vi "INTERFAZ.vi"() -> ()   [LabVIEW 2017]
uses:
  <vilib>/Instr/_visa.llb/VISA Configure Serial Port (Instr).vi
panel:
  out "V1 / V2":dbl
  out "Q 2  [m3/s] 2":dbl
  out "V2  [m3/s] 2":dbl
  out "V1  [m/s] 2":dbl
  out "Q 1 [m3/s] 2":dbl
  out "Q 2  [m3/s]":dbl
  out "P2 [Pa]":dbl
  out "P1  [Pa]":dbl
  out "V2  [m/s]":dbl
  out "V1  [m/s]":dbl
  out "Q 1 [m3/s]":dbl
  out "P1 / P2":dbl
  in  "ELECTROVALVULA":bool
  out "BYTE 7":u8
  out "BYTE 6":u8
  out "BYTE 5":u8
  out "BYTE 4":u8
  out "BYTE 3":u8
  out "BYTE 2":u8
  out "BYTE 1":u8
  out "BYTE0":u8
  in  "PUERTO SERIE ARDUINO":refnum<visa-resource-name>
  in  "STOP":bool
  out "CAUDAL 2 [L/min]":dbl(knob) scale=0.0..800.0
  out "CAUDAL 1 [L/min]":dbl(knob) scale=0.0..800.0
  out "PRESION 1 [PSI]":dbl(knob) scale=10.0..80.0
  out "PRESION 2 [PSI]":dbl(knob) scale=10.0..80.0
  # "PROYECTO TUBO VENTURI - DEMOSTRACION EXPERIMENTAL"
  # "ERROR %"
  # "VALORES EXPERIMENTALES"
  # "VALORES TEORICOS"
  # "RELACIONES"
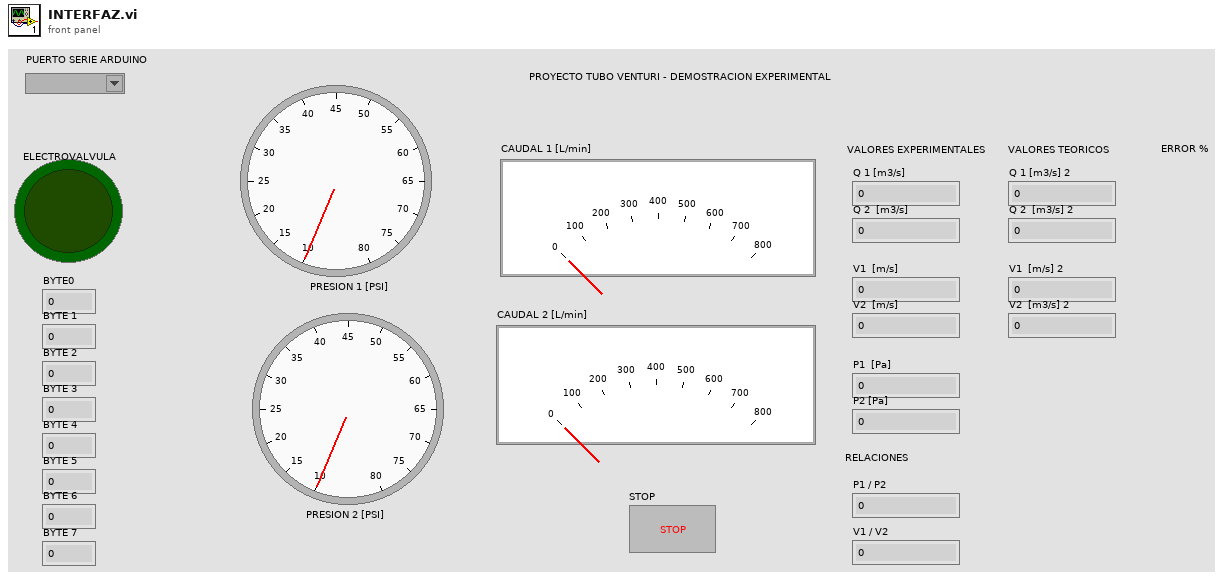
[diagram p1: front panel]
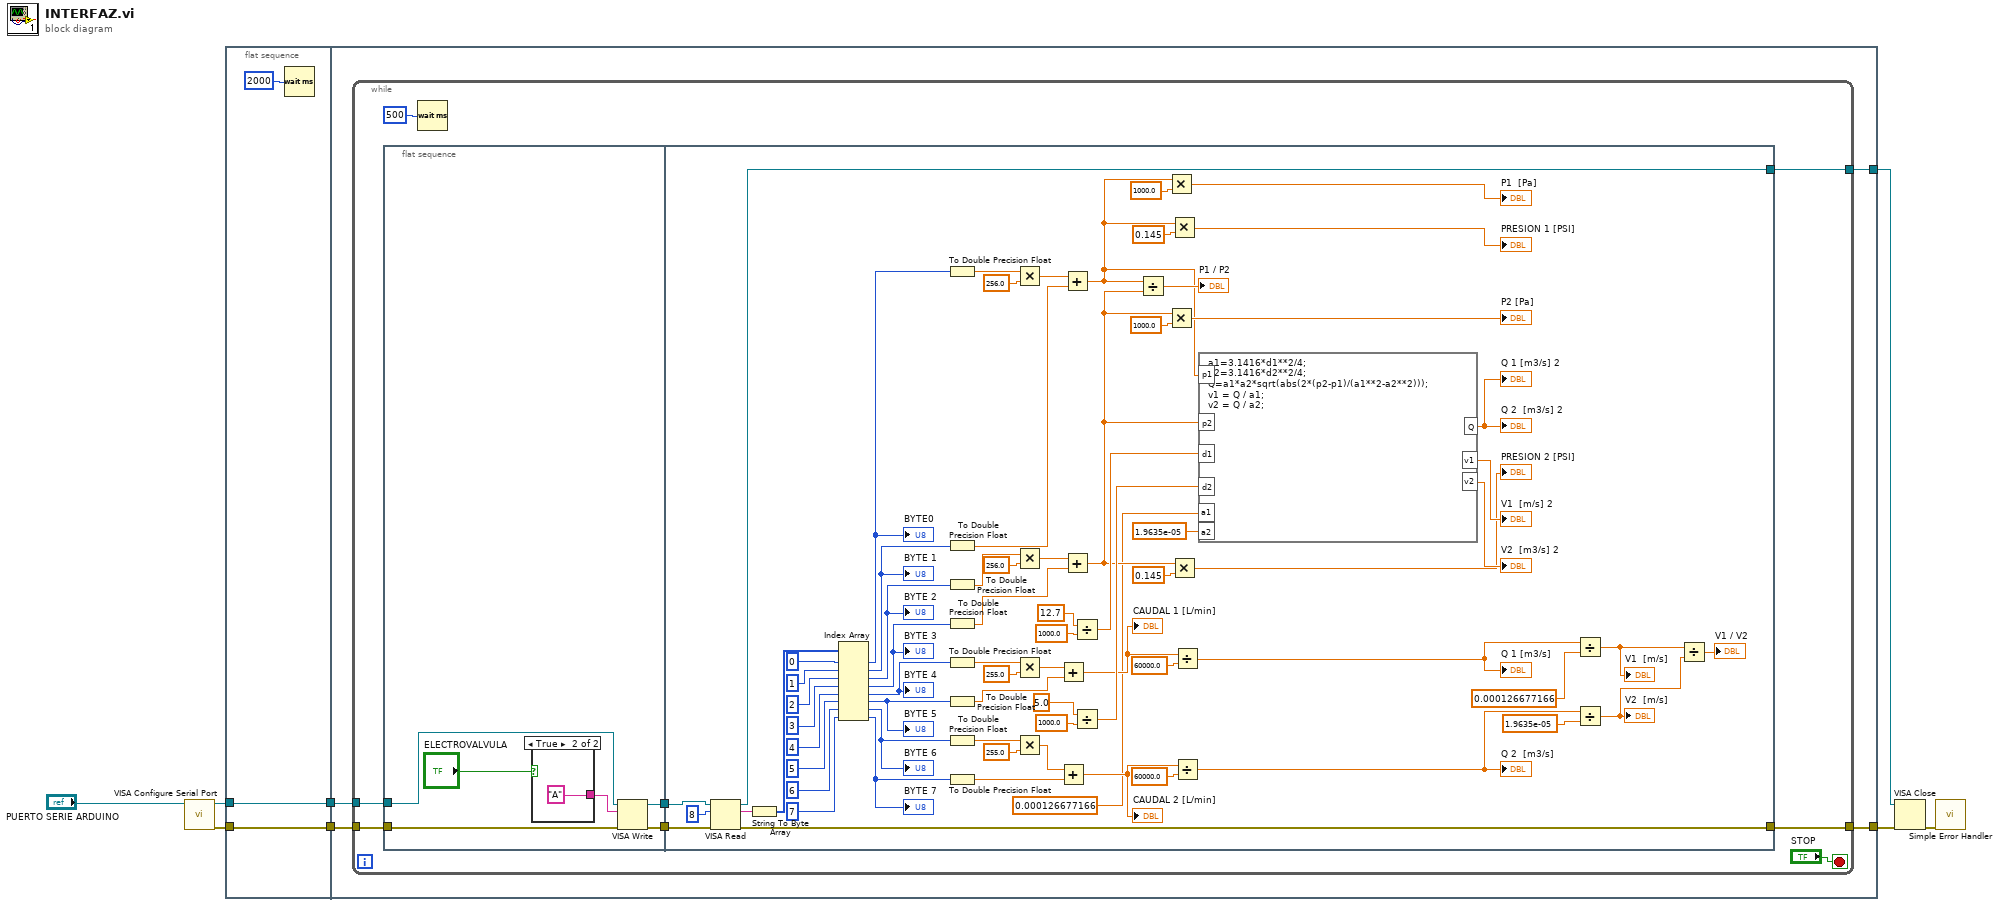
[diagram p0: block diagram]
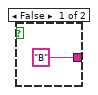
[diagram p2: hidden frame]
diagram:
  n1 = call-poly "VISA Configure Serial Port"("VISA resource name"="PUERTO SERIE ARDUINO") -> ("VISA resource name out"=w6:refnum<visa-resource-name>, "error out"=w4:errorcluster)  [unwired: 13 in]
  n2 = flat-sequence {
    tunnel: [w10] -> w7
    tunnel: w6 -> [w10]
    tunnel: [w9] -> w5
    tunnel: w4 -> [w9]
    tunnel: w7 -> [w14]
    tunnel: w5 -> [w15]
    tunnel: [w13] -> w3
    tunnel: [w12] -> w2
    frame #0 {
      n3 = Wait (ms)(milliseconds to wait=u32 2000) -> ()  [unwired: 1 out]
    }
    frame #1 {
      n4 = while {
        tunnel: w15 -> [w22]
        tunnel: w14 -> [w21]
        tunnel: [w18] -> w13
        tunnel: [w17] -> w12
        stop <- "STOP" stop-if-true
        n5 = flat-sequence {
          tunnel: w22 -> [w29]
          tunnel: w21 -> [w28]
          tunnel: [w27] -> w20
          tunnel: [w26] -> w19
          tunnel: w20 -> [w103]
          tunnel: w19 -> [w102]
          tunnel: [w96] -> w18
          tunnel: [w95] -> w17
          frame #0 {
            n6 = case shown="True" "ELECTROVALVULA" {
              tunnel: ["B" ("write buffer") "A" ("write buffer")] -> w24
              frame False {
              }
              frame True {
              }
            }
            n7 = VISA Write(VISA resource name=w28, write buffer=w24, error in (no error)=w29) -> (VISA resource name out=w27:refnum<visa-resource-name>, error out=w26:errorcluster)  [unwired: 1 out]
          }
          frame #1 {
            n8 = VISA Read(VISA resource name=w103, byte count=u32 8, error in (no error)=w102) -> (VISA resource name out=w96:refnum<visa-resource-name>, read buffer=w100:string, error out=w95:errorcluster)  [unwired: 1 out]
            n9 = String To Byte Array(string=w100) -> (unsigned byte array=w99:u8[])
            n10 = Index Array(array=w99, index #1=0 ("index"), index #2=1 ("index"), index #3=2 ("index"), index #4=3 ("index"), index #5=4 ("index"), index #6=5 ("index"), index #7=6 ("index"), index #8=7 ("index")) -> (element #1=w85:u8, element #2=w83:u8, element #3=w78:u8, element #4=w77:u8, element #5=w72:u8, element #6=w71:u8, element #7=w66:u8, element #8=w65:u8)
            "BYTE0" <- w85
            "BYTE 1" <- w83
            "BYTE 2" <- w78
            "BYTE 3" <- w77
            "BYTE 4" <- w72
            "BYTE 5" <- w71
            "BYTE 6" <- w66
            "BYTE 7" <- w65
            n11 = To Double Precision Float(number=w85) -> (double precision float=w86:dbl)
            n12 = To Double Precision Float(number=w83) -> (double precision float=w84:dbl)
            n13 = To Double Precision Float(number=w78) -> (double precision float=w80:dbl)
            n14 = To Double Precision Float(number=w77) -> (double precision float=w79:dbl)
            n15 = To Double Precision Float(number=w72) -> (double precision float=w74:dbl)
            n16 = To Double Precision Float(number=w71) -> (double precision float=w73:dbl)
            n17 = To Double Precision Float(number=w66) -> (double precision float=w68:dbl)
            n18 = To Double Precision Float(number=w65) -> (double precision float=w67:dbl)
            n19 = Multiply(x=w86, y=256.0) -> (x*y=w87:dbl)
            n20 = Multiply(x=w80, y=256.0) -> (x*y=w81:dbl)
            n21 = Multiply(x=w74, y=255.0) -> (x*y=w75:dbl)
            n22 = Multiply(x=w68, y=255.0) -> (x*y=w69:dbl)
            n23 = Add(x=w75, y=w73) -> (x+y=w53:dbl)
            "CAUDAL 1 [L/min]" <- w53
            n24 = Add(x=w69, y=w67) -> (x+y=w50:dbl)
            "CAUDAL 2 [L/min]" <- w50
            n25 = Add(x=w87, y=w84) -> (x+y=w41:dbl)
            n26 = Add(x=w81, y=w79) -> (x+y=w45:dbl)
            n27 = Divide(x=12.7 ("input variable"), y=1000.0) -> (x/y=w59:dbl)
            n28 = Divide(x=5.0 ("input variable"), y=1000.0) -> (x/y=w58:dbl)
            n29 = Divide(x=w41, y=w45) -> (x/y=→"P1 / P2":dbl)
            n30 = Multiply(x=w41, y=1000.0) -> (x*y=→"P1  [Pa]":dbl)
            n31 = Multiply(x=w45, y=1000.0) -> (x*y=→"P2 [Pa]":dbl)
            n32 = Multiply(x=w41, y=0.145) -> (x*y=→"PRESION 1 [PSI]":dbl)
            n33 = Multiply(x=w45, y=0.145) -> (x*y=→"PRESION 2 [PSI]":dbl)
            n34 = Divide(x=w53, y=60000.0) -> (x/y=w38:dbl)
            "Q 1 [m3/s]" <- w38
            n35 = Divide(x=w50, y=60000.0) -> (x/y=w35:dbl)
            "Q 2  [m3/s]" <- w35
            n36 = formula code="a1=3.1416*d1**2/4;\na2=3.1416*d2**2/4;\nQ=a1*a2*sqrt(abs(2*(p2-p1)/(a1**2-a2**2)));\nv1 = Q / a1;\nv2 = Q / a2;"("p1"=w41, "p2"=w45, "d1"=w59, "d2"=w58, "a1"=0.000126677166 ("input variable"), "a2"=1.9635e-05 ("input variable")) -> ("Q"=→"Q 1 [m3/s] 2" →"Q 2  [m3/s] 2":dbl, "v1"=→"V1  [m/s] 2":dbl, "v2"=→"V2  [m3/s] 2":dbl)
            n37 = Divide(x=w38, y=0.000126677166) -> (x/y=w33:dbl)
            "V1  [m/s]" <- w33
            n38 = Divide(x=w35, y=1.9635e-05) -> (x/y=w32:dbl)
            "V2  [m/s]" <- w32
            n39 = Divide(x=w33, y=w32) -> (x/y=→"V1 / V2":dbl)
          }
        }
        n40 = Wait (ms)(milliseconds to wait=u32 500) -> ()  [unwired: 1 out]
      }
    }
  }
  n41 = VISA Close(VISA resource name=w3, error in (no error)=w2) -> (error out=w1:errorcluster)
  n42 = call <vilib>:"Simple Error Handler.vi"("error in (no error)"=w1) -> ()  [unwired: 4 in, 5 out]
